vi "deleteEmplProjet.vi"(0 "id projet":string, 1 "Id Personnel":string, 2 "OK Button":bool) -> ()   [LabVIEW 2024]
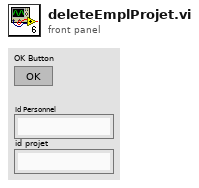
[diagram p1: front panel]
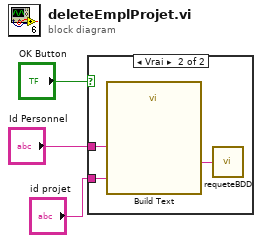
[diagram p0: block diagram]
diagram:
  n1 = case shown="Vrai" "OK Button" {
    tunnel: "Id Personnel" -> [_ w6]
    tunnel: "id projet" -> [_ w4]
    frame False {
    }
    frame True {
      n2 = call "Build Text"("id_persoonel"=w6, "id_projet"=w4) -> ("Result"=w5:string)  [unwired: 12 in, 1 out]
      n3 = call "requeteBDD.vi"("Requête Sql"=w5) -> ()  [unwired: 1 out]
    }
  }
